vi "local_linear_smooth_double_1d.vi"(1 "Smoothing Parameter (Gaussian S.D. in pixels)":dbl=3.0, 2 "Input Array":dbl[](graph)) -> (0 "Smoothed Array":dbl[](graph))   [LabVIEW 2010]
uses:
  <vilib>/Analysis/baseanly.llb/A x Vector.vi
  <vilib>/Analysis/NI_AALBase.lvlib
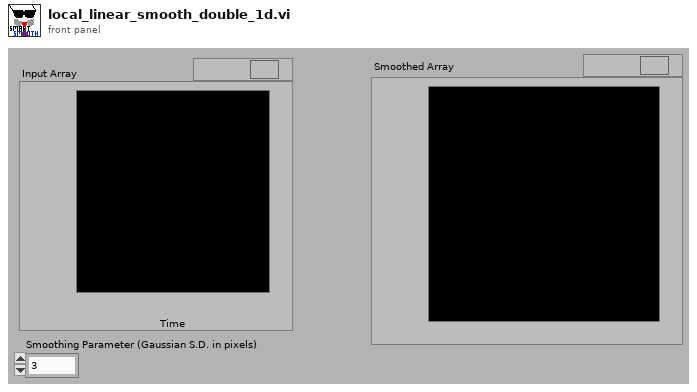
[diagram p1: front panel]
types:
  T1 = cluster{"Smoothing Parameter (Gaussian S.D. in pixels)":dbl, i32}
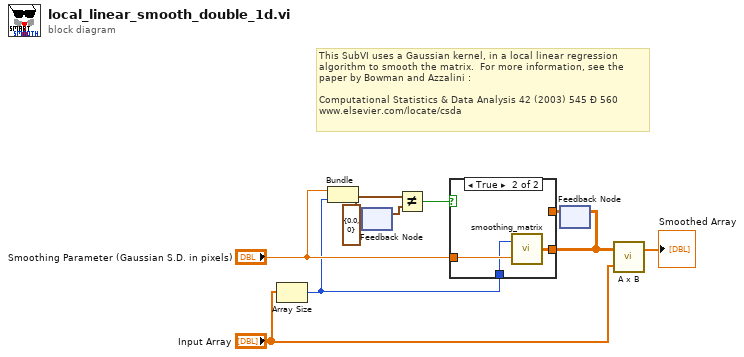
[diagram p0: block diagram]
diagram:
  # "This SubVI uses a Gaussian kernel, in a local linear regression algorithm to smooth the matrix.  For more information, see the paper by Bowman and Azzalini :\n\nComputational Statistics & Data Analysis 42 (2003) 545 Ð 560 \nwww.elsevier.com/locate/csda"
  n1 = Array Size(array="Input Array") -> (size(s)=w5:i32)
  n2 = Bundle("Smoothing Parameter (Gaussian S.D. in pixels)"="Smoothing Parameter (Gaussian S.D. in pixels)", w5) -> (w7:T1)  [unwired: 1 out]
  n3 = feedback-in #1(w7) -> ()
  n4 = feedback #1(T1 {"Smoothing Parameter (Gaussian S.D. in pixels)"=0.0, 0}) -> (w8:T1)
  n5 = Not Equal?(x=w7, y=w8) -> (x != y?=w3:bool)
  n6 = feedback #2() -> (w1:dbl[][])  [unwired: 1 out]
  n7 = case shown="True" w3 {
    tunnel: [w11 w14] -> w2
    tunnel: "Smoothing Parameter (Gaussian S.D. in pixels)" -> [_ w13]
    tunnel: w5 -> [_ w12]
    tunnel: w1 -> [w11 _]
    frame False {
    }
    frame True {
      n8 = call "smoothing_matrix.vi"("Smoothing Parameter (Gaussian S.D. in pixels)"=w13, "Size"=w12) -> ("Smoothing Matrix"=w14:dbl[][])
    }
  }
  n9 = feedback-in #2(w2) -> ()
  n10 = call-poly <vilib>:"A x B.vi"("Vector"="Input Array", "A"=w2) -> ("A x Vector"=→"Smoothed Array":dbl[])  [unwired: 1 out]
